vi "Poke and Probe Right.vi"(4 "Tap In?":bool, 6 "Release Part":bool=TRUE, 7 "Goal":T1={"X"=603.7814077996513, "Y"=-344.17047969163804, "Z"=12.0, "O"=0.0, "A"=0.0, "T"=0.0}, 8 "error in":errorcluster, 11 "Location":string="Base") -> (0 "error out":errorcluster, 3 "Location Out":string=" ", 5 "time":dbl=15.3)   [LabVIEW 2013]
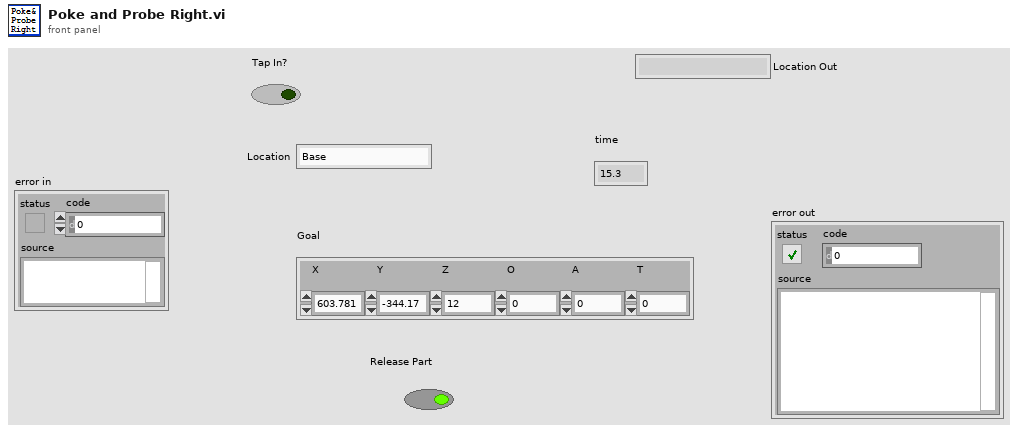
[diagram p1: front panel]
types:
  T1 = cluster{"X":dbl, "Y":dbl, "Z":dbl, "O":dbl, "A":dbl, "T":dbl}
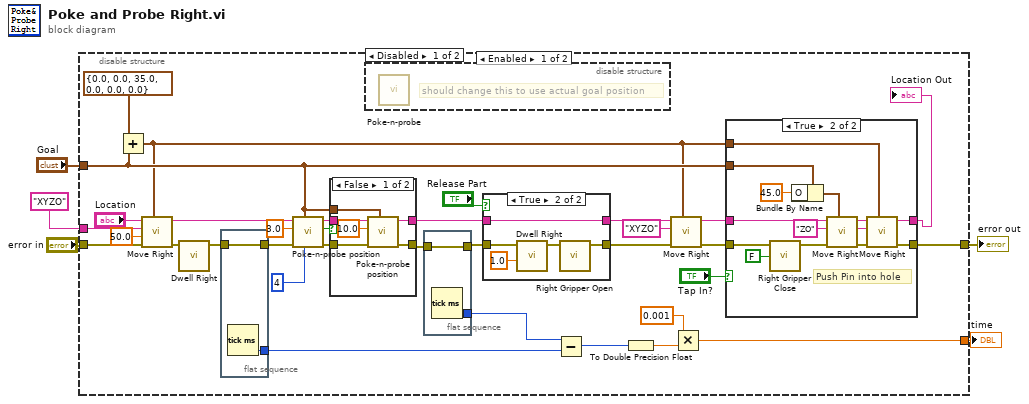
[diagram p0: block diagram]
diagram:
  n1 = disable-structure shown="Enabled" {
    disable-tunnel: [w9 _] -> w5
    disable-tunnel: [w28 _] -> w4
    disable-tunnel: "Goal" -> [w11 _]
    disable-tunnel: "error in" -> [w21 _]
    disable-tunnel: "XYZO" ("Mask") -> [w20 _]
    frame Enabled {
      n2 = Add(x=T1 {"X"=0.0, "Y"=0.0, "Z"=35.0, "O"=0.0, "A"=0.0, "T"=0.0} ("Goal Axes"), y=w11) -> (x+y=w8:T1)
      n3 = call "Move Right.vi"("Goal"=w8, "error in"=w21, "Speed"=50.0, "Mask"=w20, "Location"="Location") -> ("error out"=w19:errorcluster, "Location Out"=w13:string)  [unwired: 2 in, 3 out]
      n4 = call "Dwell Right.vi"("error in"=w19) -> ("error out"=w18:errorcluster)  [unwired: 10 in]
      n5 = flat-sequence {
        tunnel: [w59] -> w23
        tunnel: w18 -> [w58]
        tunnel: [w58] -> w27
        frame #0 {
          n6 = Tick Count (ms)() -> (millisecond timer value=w59:u32)
        }
      }
      n7 = call "Poke-n-probe position.vi"("Tries"=4, "Goal"=w11, "error in"=w27, "Zone"=3.0, "Location"=w13) -> ("error out"=w34:errorcluster, "Success"=w35:bool, "Location Out"=w16:string)  [unwired: 2 in, 2 out]
      n8 = case shown="False" w35 {
        tunnel: w11 -> [w72 _]
        tunnel: w34 -> [w70 w74]
        tunnel: [w69 w74] -> w25
        tunnel: w16 -> [w68 w73]
        tunnel: [w67 w73] -> w15
        frame False {
          n9 = call "Poke-n-probe position.vi"("Goal"=w72, "error in"=w70, "Zone"=10.0, "Location"=w68) -> ("error out"=w69:errorcluster, "Location Out"=w67:string)  [unwired: 3 in, 3 out]
        }
        frame True {
        }
      }
      n10 = disable-structure shown="Disabled" {
        frame Disabled {
          # "should change this to use actual goal position"
          n11 = call "Poke-n-probe.vi"() -> ()  [unwired: 7 in, 5 out]
        }
        frame Enabled {
        }
      }
      n12 = flat-sequence {
        tunnel: [w57] -> w24
        tunnel: w25 -> [w56]
        tunnel: [w56] -> w26
        frame #0 {
          n13 = Tick Count (ms)() -> (millisecond timer value=w57:u32)
        }
      }
      n14 = case shown="True" "Release Part" {
        tunnel: [w61 w66] -> w38
        tunnel: w26 -> [w61 w64]
        tunnel: w15 -> [w60 w62]
        tunnel: [w60 w62] -> w14
        frame False {
        }
        frame True {
          n15 = call "Dwell Right.vi"("Wait Time"=1.0, "error in"=w64) -> ("error out"=w63:errorcluster)  [unwired: 9 in]
          n16 = call "Right Gripper Open.vi"("error in"=w63) -> ("error out"=w66:errorcluster)  [unwired: 10 in]
        }
      }
      n17 = Subtract(x=w24, y=w23) -> (x-y=w22:u32)
      n18 = To Double Precision Float(number=w22) -> (double precision float=w29:dbl)
      n19 = call "Move Right.vi"("Goal"=w8, "error in"=w38, "Mask"="XYZO", "Location"=w14) -> ("error out"=w39:errorcluster, "Location Out"=w10:string)  [unwired: 3 in, 3 out]
      n20 = Multiply(x=0.001 ("y"), y=w29) -> (x*y=w28:dbl)
      n21 = case shown="True" "Tap In?" {
        tunnel: w39 -> [w40 w55]
        tunnel: w11 -> [_ w44]
        tunnel: w10 -> [w41 w51]
        tunnel: [w40 w49] -> w9
        tunnel: w8 -> [_ w48]
        tunnel: [w41 w45] -> w7
        frame False {
        }
        frame True {
          # "Push Pin into hole"
          n22 = call "Right Gripper Close.vi"("Pause on Miss?"=FALSE, "error in"=w55) -> ("error out"=w53:errorcluster)  [unwired: 8 in, 1 out]
          n23 = Bundle By Name(cluster=w44, "O"=45.0) -> (w43:T1)
          n24 = call "Move Right.vi"("Goal"=w43, "error in"=w53, "Mask"="ZO", "Location"=w51) -> ("error out"=w50:errorcluster, "Mask Out"=w46:string, "Location Out"=w47:string)  [unwired: 3 in, 2 out]
          n25 = call "Move Right.vi"("Goal"=w48, "error in"=w50, "Mask"=w46, "Location"=w47) -> ("error out"=w49:errorcluster, "Location Out"=w45:string)  [unwired: 3 in, 3 out]
        }
      }
      "Location Out" <- w7
    }
    frame Disabled {
    }
  }
  "time" <- w4
  "error out" <- w5
